vi "lightfield normalization.vi"(10 "ROI array":i32[][](array[numeric])) -> (2 "ROI norm":dbl[][](array[numeric]))   [LabVIEW 2012]
uses:
  <vilib>/Analysis/NI_AALBase.lvlib
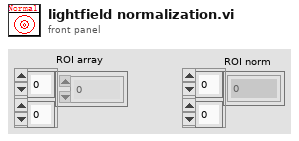
[diagram p1: front panel]
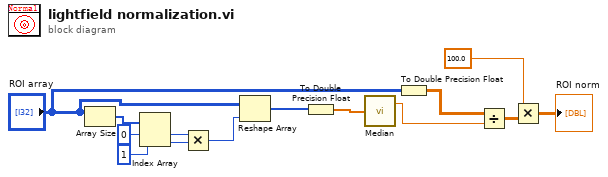
[diagram p0: block diagram]
diagram:
  n1 = Array Size(array="ROI array") -> (size(s)=w8:i32[])
  n2 = Index Array(array=w8, index #1=0 ("索引"), index #2=1 ("索引")) -> (element #1=w4:i32, element #2=w5:i32)
  n3 = Multiply(x=w4, y=w5) -> (x*y=w3:i32)
  n4 = Reshape Array("ROI array", w3) -> (w14:i32[])
  n5 = To Double Precision Float(number=w14) -> (double precision float=w13:dbl[])
  n6 = call <vilib>:"Median.vi"("X"=w13) -> ("median"=w12:dbl)  [unwired: 1 out]
  n7 = To Double Precision Float(number="ROI array") -> (double precision float=w11:dbl[][])
  n8 = Divide(x=w11, y=w12) -> (x/y=w9:dbl[][])
  n9 = Multiply(x=100.0, y=w9) -> (x*y=→"ROI norm":dbl[][])
